vi "NiFPGA Write FIFO - I32.vi"(6 "Timeout":u32, 8 "error in (no error)":errorcluster, 9 "Data":i32[](array[numeric]), 10 "FIFO":u32, 11 "Session":u32) -> (0 "error out":errorcluster, 3 "Session Out":u32, 4 "Empty Elements Remaining":u32)   [LabVIEW 2010, in "FPGA Interface Wrapper.lvlib"]
doc: "Writes to a FIFO of signed 32-bit integers."
uses:
  <userlib>/_FPGA Interface Advanced Tools/FPGA Interface Wrapper/FPGA Interface Wrapper.lvlib
  NiFpga.dll
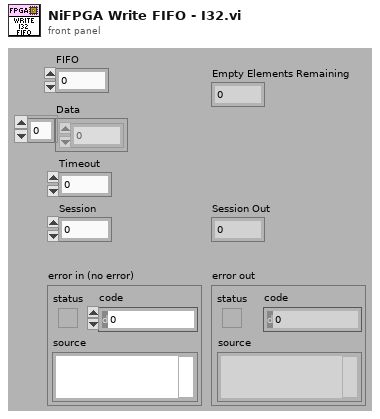
[diagram p1: front panel]
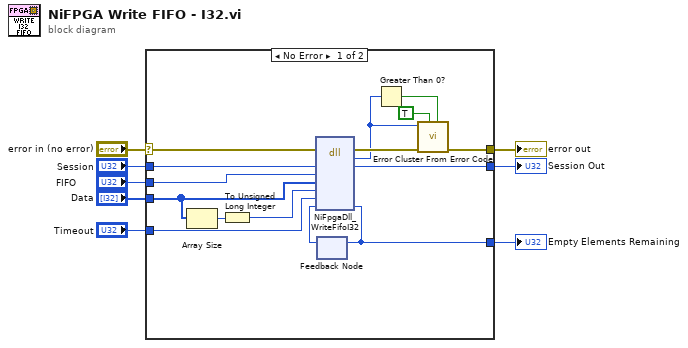
[diagram p0: block diagram]
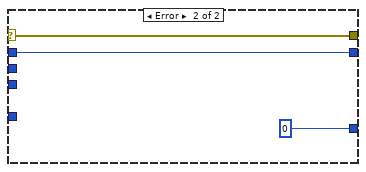
[diagram p2: hidden frame]
diagram:
  n1 = case shown="No Error" "error in (no error)" {
    selector: "error in (no error)" -> [w23 w25]
    tunnel: [w11 w25] -> w7
    tunnel: "Session" -> [w22 w26]
    tunnel: [w21 w26] -> w5
    tunnel: "FIFO" -> [w20 _]
    tunnel: "Timeout" -> [w19 _]
    tunnel: [w10 u64 0 ("Elements Remaining")] -> w2
    tunnel: "Data" -> [w16 _]
    frame No Error {
      n2 = Array Size(array=w16) -> (size(s)=w18:i32)
      n3 = To Unsigned Long Integer(number=w18) -> (unsigned 32bit integer=w17:u32)
      n4 = feedback #1() -> (w9:u64)  [unwired: 1 in]
      n5 = dll-call lib="NiFpga.dll" fn="NiFpgaDll_WriteFifoI32"(error in=w23, "Session"=w22, "FIFO"=w20, "Data"=w16, "Number of Elements"=w17, "Timeout"=w19, "Empty Elements Remaining"=w9) -> (error out=w13:errorcluster, "Status"=w12:i32, "Session"=w21:u32, "Empty Elements Remaining"=w10:u64)  [unwired: 6 in, 1 out]
      n6 = feedback-in #1(w10) -> ()
      n7 = Greater Than 0?(x=w12) -> (x > 0?=w14:bool)
      n8 = call <vilib>:"Error Cluster From Error Code.vi"("is warning? (False)"=w14, "show call chain? (False)"=TRUE, "error in (no error)"=w13, "error code (0)"=w12) -> ("error out"=w11:errorcluster)  [unwired: 5 in]
    }
    frame Error {
    }
  }
  "error out" <- w7
  "Session Out" <- w5
  "Empty Elements Remaining" <- w2
